vi "Twiddle Address Generator.vi"(2 "Reset?":bool, 3 "Address Type":T1, 7 "Increment?":bool) -> (8 "Twiddle Address":T2 format="%.21g")   [LabVIEW 2011]
uses:
  BRAM Phase FXP Type.ctl
  Twiddle Address FXP Type.ctl
  <vilib>/rvi/FXPMathLib/FxpInterpret/XNode/nifxpmath_Interpret.xnode
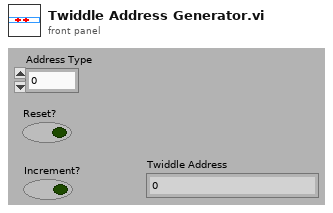
[diagram p1: front panel]
types:
  T1 = typedef "Twiddle Address FXP Type.ctl" = fxp<+,9,9>
  T2 = typedef "BRAM Phase FXP Type.ctl" = fxp<+/-,14,1>
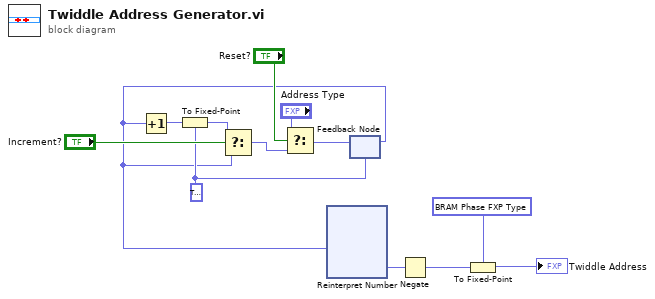
[diagram p0: block diagram]
diagram:
  w6 = T1 0.0 ("Counter FXP Type")
  n1 = feedback #1(w6) -> (w5:T1)
  n2 = Increment(x=w5) -> (x+1=w13:fxp<+,10,10>)
  n3 = To Fixed-Point(fixed-point type=w6, number=w13) -> (fixed-point=w12:T1)
  n4 = Select(t=w12, s="Increment?", f=w5) -> (s? t:f=w9:T1)
  n5 = Select(t="Address Type", s="Reset?", f=w9) -> (s? t:f=w7:T1)
  n6 = xnode "Reinterpret Number"("x"=w5) -> ("y"=w4:fxp<+,9,0>)
  n7 = feedback-in #1(w7) -> ()
  n8 = Negate(x=w4) -> (-x=w2:fxp<+/-,10,1>)
  n9 = To Fixed-Point(fixed-point type=T2 0.0, number=w2) -> (fixed-point=→"Twiddle Address":T2)
